vi "I2C communication.vi"() -> ()   [LabVIEW 2019]
doc: "I2C communication allows a user to select the addressing scheme, to read or write to a device, and the mode (standard or fast) to execute the data communication."
uses:
  <vilib>/eio/EIONode/EIONode.xnode
panel:
  in  "Receiver Address":u8 format="%b"
  in  "Addressing Scheme":i16(ring)=7 items=["7-bit address", "10-bit address"]
  out "Data bit array":bool[](array[boolean])
  in  "Number of Bytes":i16
  in  "Data to send":u8[](array[numeric])=[0, 0] format="%b"
  in  "Read/Write?":bool
  in  "Mode":i16(ring) items=["Standard ", "Fast", "High-Speed"]
  in  "Start\nSending":bool
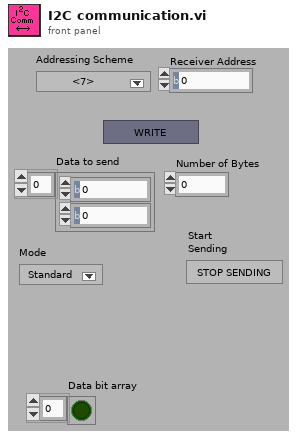
[diagram p1: front panel]
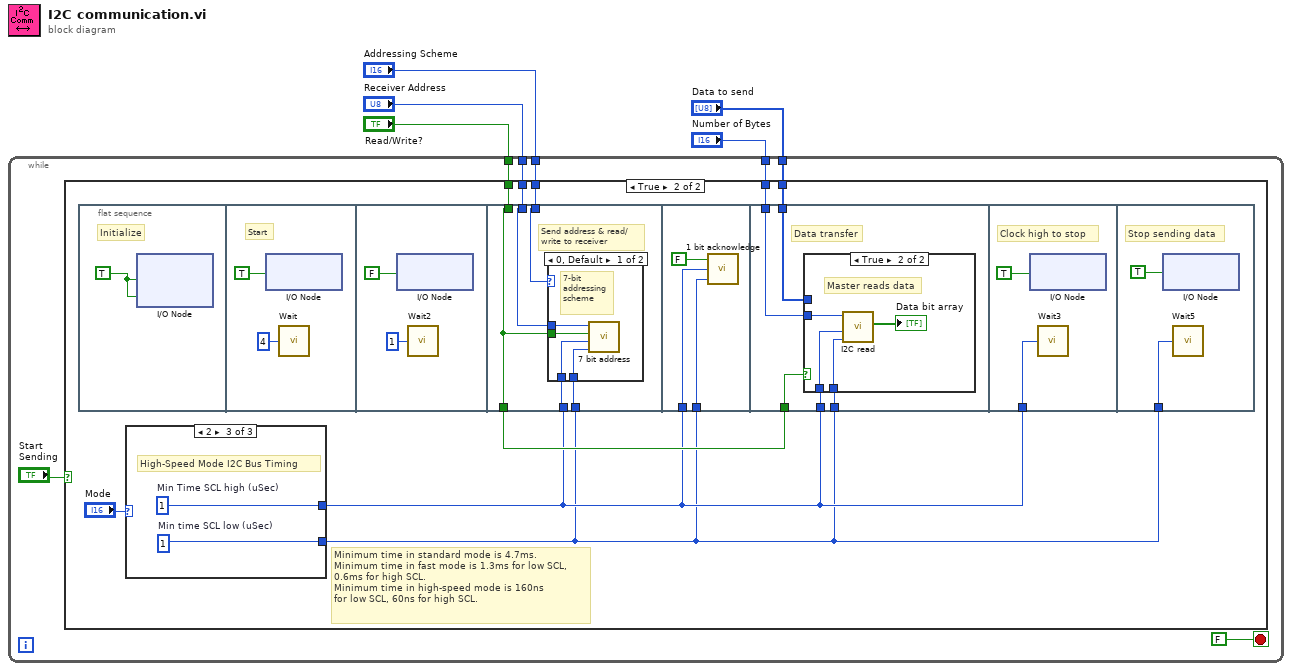
[diagram p0: block diagram]
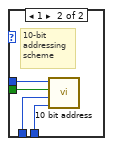
[diagram p3: hidden frame]
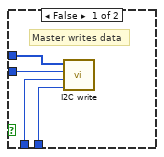
[diagram p4: hidden frame]
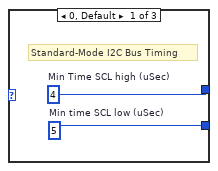
[diagram p5: hidden frame]
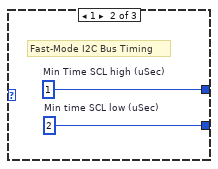
[diagram p6: hidden frame]
diagram:
  n1 = while {
    tunnel: "Addressing Scheme" -> [w12]
    tunnel: "Receiver Address" -> [w11]
    tunnel: "Read/Write?" -> [w10]
    tunnel: "Data to send" -> [w9]
    tunnel: "Number of Bytes" -> [w8]
    stop <- FALSE stop-if-true
    n2 = case shown="True" "Start\nSending" {
      tunnel: w12 -> [_ w21]
      tunnel: w11 -> [_ w20]
      tunnel: w10 -> [_ w19]
      tunnel: w9 -> [_ w18]
      tunnel: w8 -> [_ w17]
      frame False {
      }
      frame True {
        # "Minimum time in standard mode is 4.7ms.\nMinimum time in fast mode is 1.3ms for low SCL,\n0.6ms for high SCL.\nMinimum time in high-speed mode is 160ns \nfor low SCL, 60ns for high SCL."
        n3 = flat-sequence {
          tunnel: [w27] -> w16
          tunnel: w15 -> [w31]
          tunnel: w14 -> [w30]
          tunnel: w21 -> [w29]
          tunnel: w20 -> [w28]
          tunnel: w19 -> [w27]
          tunnel: w15 -> [w41]
          tunnel: w14 -> [w40]
          tunnel: w16 -> [w47]
          tunnel: w15 -> [w46]
          tunnel: w14 -> [w45]
          tunnel: w18 -> [w44]
          tunnel: w17 -> [w43]
          tunnel: w15 -> [w56]
          tunnel: w14 -> [w59]
          frame #0 {
            w22 = TRUE ("Digital Out")
            # "Initialize"
            n4 = xnode "I/O Node"("SDA"=w22, "SCL"=w22) -> ()  [unwired: 2 in, 2 out]
          }
          frame #1 {
            # "Start"
            n5 = xnode "I/O Node"("SDA"=TRUE ("Start Sending")) -> ()  [unwired: 1 in, 1 out]
            n6 = call "Wait"("Count(uSec)"=u32 4) -> ()  [unwired: 1 out]
          }
          frame #2 {
            n7 = xnode "I/O Node"("SCL"=FALSE ("Digital Out")) -> ()  [unwired: 1 in, 1 out]
            n8 = call "Wait2"("Count(uSec)"=u32 1) -> ()  [unwired: 1 out]
          }
          frame #3 {
            # "Send address & read/write to receiver"
            n9 = case shown="0, Default" w29 {
              tunnel: w28 -> [w35 w39]
              tunnel: w27 -> [w34 w38]
              tunnel: w31 -> [w33 w37]
              tunnel: w30 -> [w32 w36]
              frame 0, Default {
                # "7-bit addressing scheme"
                n10 = call "7 bit address.vi"("Min time SCL low (uSec)"=w32, "Min Time SCL high (uSec)"=w33, "Read/Write?"=w34, "Receiver Address"=w35) -> ()
              }
              frame 1 {
                # "10-bit addressing scheme"
                n11 = call "10 bit address.vi"("Min time SCL low (uSec)"=w36, "Min Time SCL high (uSec)"=w37, "Read/Write?"=w38, "Receiver Address"=w39) -> ()
              }
            }
          }
          frame #4 {
            n12 = call "1 bit acknowledge.vi"("Min time SCL low (uSec)"=w40, "Min Time SCL high (uSec)"=w41, "Acknowledgement"=FALSE) -> ()
          }
          frame #5 {
            # "Data transfer"
            n13 = case shown="True" w47 {
              tunnel: w44 -> [w51 _]
              tunnel: w43 -> [w50 w55]
              tunnel: w46 -> [w49 w53]
              tunnel: w45 -> [w48 w52]
              frame False {
                # "Master writes data"
                n14 = call "I2C write.vi"("Min time SCL low (uSec)"=w48, "Min Time SCL high (uSec)"=w49, "Number of Bytes"=w50, "Data to send"=w51) -> ()
              }
              frame True {
                # "Master reads data"
                n15 = call "I2C read.vi"("Min time SCL low (uSec)"=w52, "Min Time SCL high (uSec)"=w53, "Number of Bytes"=w55) -> ("Data bit array"=→"Data bit array":bool[])
              }
            }
          }
          frame #6 {
            # "Clock high to stop"
            n16 = xnode "I/O Node"("SCL"=TRUE ("Digital Out")) -> ()  [unwired: 1 in, 1 out]
            n17 = call "Wait3"("Count(uSec)"=w56) -> ()  [unwired: 1 out]
          }
          frame #7 {
            # "Stop sending data"
            n18 = xnode "I/O Node"("SDA"=TRUE ("Digital Out")) -> ()  [unwired: 1 in, 1 out]
            n19 = call "Wait5"("Count(uSec)"=w59) -> ()  [unwired: 1 out]
          }
        }
        n20 = case shown="2" "Mode" {
          tunnel: [w61 w63 w65] -> w15
          tunnel: [w60 w62 w64] -> w14
          frame 0, Default {
            w61 = 4  # Min Time SCL high (uSec)
            w60 = 5  # Min time SCL low (uSec)
            # "Standard-Mode I2C Bus Timing"
          }
          frame 1 {
            w63 = 1  # Min Time SCL high (uSec)
            w62 = 2  # Min time SCL low (uSec)
            # "Fast-Mode I2C Bus Timing"
          }
          frame 2 {
            w65 = 1  # Min Time SCL high (uSec)
            w64 = 1  # Min time SCL low (uSec)
            # "High-Speed Mode I2C Bus Timing"
          }
        }
      }
    }
  }
